vi "Calculate Elapsed Time.vi"(11 "UI Data In":T1) -> (2 "Elapsed":dbl, 3 "UI Data":T1)   [LabVIEW 2020]
doc: "Calculates the elapsed time based on the current running state, accumulated time for pauses, and the current segment time."
uses:
  controls/UI Data.ctl
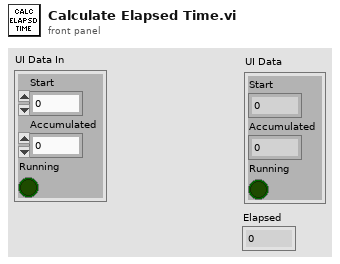
[diagram p1: front panel]
types:
  T1 = typedef "UI Data.ctl" = cluster{"Start":dbl, "Accumulated":dbl, "Running":bool}
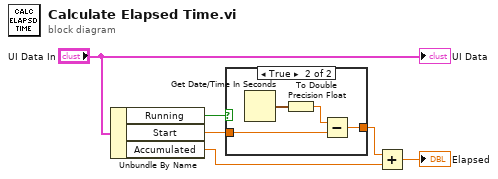
[diagram p0: block diagram]
diagram:
  n1 = Unbundle By Name("UI Data In") -> ("Running"=w1:bool, "Start"=w5:dbl, "Accumulated"=w3:dbl)
  n2 = case shown="True" w1 {
    tunnel: w5 -> [_ w9]
    tunnel: [_ w7] -> w4
    frame False {
    }
    frame True {
      n3 = Get Date/Time In Seconds() -> (seconds since 1Jan1904=w10:timestamp)
      n4 = To Double Precision Float(number=w10) -> (double precision float=w8:dbl)
      n5 = Subtract(x=w8, y=w9) -> (x-y=w7:dbl)
    }
  }
  n6 = Add(x=w4, y=w3) -> (x+y=→"Elapsed":dbl)
  "UI Data" <- "UI Data In"
